vi "Set Many Attributes Priv.vi"(0 "Tree Dictionary Out":variant, 5 "Unique ID":string, 7 "Name":string[](array[string]), 9 "Data":variant[](array[variant]), 11 "error in":errorcluster) -> (4 "Tree Dictionary Out":variant, 8 "Replaced?":bool[](array[boolean]), 15 "error out":errorcluster)   [LabVIEW 2020, in "NI_VIAnCFGDataStructure.lvlib" / "Tree.lvclass"]
uses:
  <vilib>/addons/analyzer/VIAnCFGDataStructure/Tree Manager/Tree.lvclass
  <vilib>/addons/analyzer/VIAnCFGDataStructure/Tree Manager/Typedefs/Tree Cluster.ctl
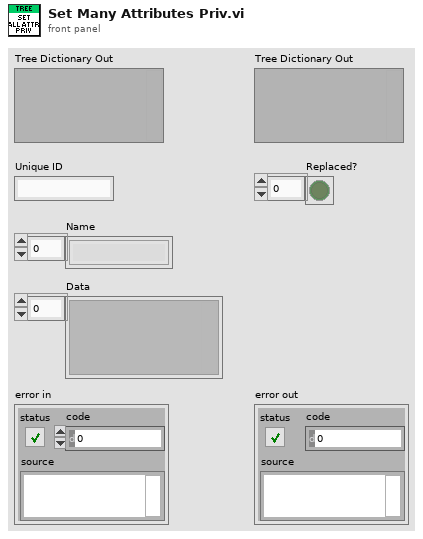
[diagram p1: front panel]
types:
  T1 = typedef "NI_VIAnCFGDataStructure.lvlib/Tree.lvclass/Tree Cluster.ctl" = cluster{"Unique ID":string, "Parent ID":string, "Child IDs":string[], "Name":string, "MetaData":string, "Data IDs":string[]}
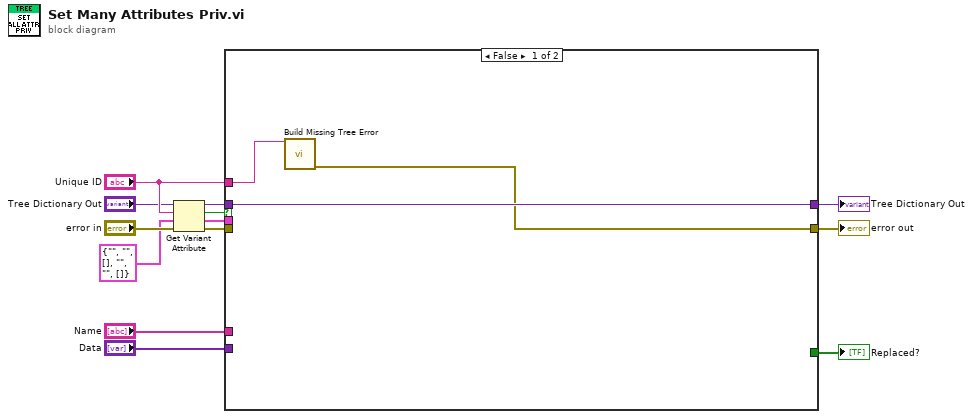
[diagram p0: block diagram]
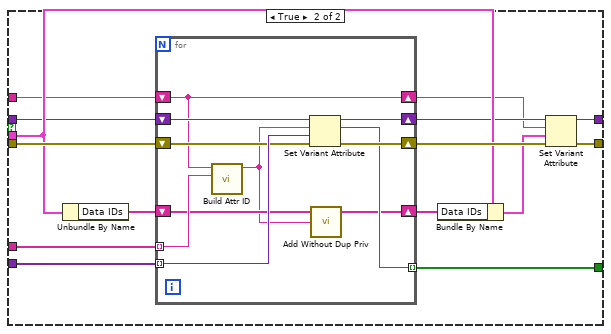
[diagram p2: hidden frame]
diagram:
  n1 = Get Variant Attribute(Variant="Tree Dictionary Out", name="Unique ID", default value (empty Variant)=T1 {"Unique ID"="", "Parent ID"="", "Child IDs"=[], "Name"="", "MetaData"="", "Data IDs"=[]} ("Cluster of class private data"), error in="error in") -> (duplicate Variant=w9:variant, found=w10:bool, value=w11:T1, error out=w7:errorcluster)
  n2 = case shown="False" w10 {
    tunnel: [w14 w31] -> w5
    tunnel: [w16 w30] -> w6
    tunnel: w7 -> [_ w28]
    tunnel: w9 -> [w16 w21]
    tunnel: w11 -> [_ w26]
    tunnel: "Name" -> [_ w23]
    tunnel: "Data" -> [_ w29]
    tunnel: "Unique ID" -> [w15 w20]
    tunnel: [_ w24] -> w3
    frame False {
      n3 = call <vilib>:"Build Missing Tree Error.vi"("Unique ID"=w15) -> ("Error Out"=w14:errorcluster)  [unwired: 14 in]
    }
    frame True {
      n4 = Unbundle By Name(w26) -> ("Data IDs"=w18:string[])
      n5 = for {
        tunnel: w29 -> [w41] mode=indexing
        tunnel: w23 -> [w35] mode=indexing
        tunnel: [w37] -> w24 mode=indexing
        shift-right: [w39] -> w27
        shift-left: w28 -> [w40]
        shift-right: [w42] -> w22
        shift-left: w21 -> [w38]
        shift-right: [w36] -> w19
        shift-left: w20 -> [w36]
        shift-right: [w32] -> w17
        shift-left: w18 -> [w34]
        n6 = call <vilib>:"Build Attr ID.vi"("Attr Name"=w35, "Unique ID"=w36) -> ("Attr ID Out"=w33:string)  [unwired: 9 in]
        n7 = Set Variant Attribute(Variant=w38, name=w33, value=w41, error in=w40) -> (Variant out=w42:variant, replaced=w37:bool, error out=w39:errorcluster)
        n8 = call <vilib>:"Add Without Dup Priv.vi"("Add String"=w33, "Strings In"=w34) -> ("Strings Out"=w32:string[])  [unwired: 3 in]
      }
      n9 = Bundle By Name(cluster=w26, "Data IDs"=w17) -> (w25:T1)
      n10 = Set Variant Attribute(Variant=w22, name=w19, value=w25, error in=w27) -> (Variant out=w30:variant, error out=w31:errorcluster)  [unwired: 1 out]
    }
  }
  "Tree Dictionary Out" <- w6
  "error out" <- w5
  "Replaced?" <- w3
